vi "SubVI_GetIterNum.vi"(1 "#iter outer loop":i32, 2 "#iter inner loop":i32[](array[numeric]), 3 "N inner loop":i32) -> (0 "#iter GLOBAL":i32[](array[numeric]))   [LabVIEW 2018]
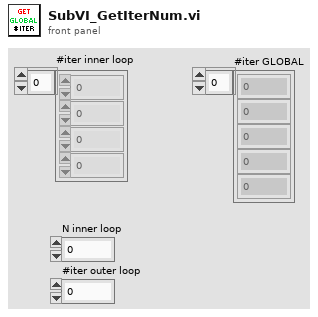
[diagram p1: front panel]
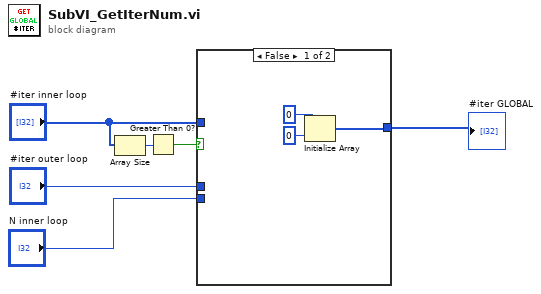
[diagram p0: block diagram]
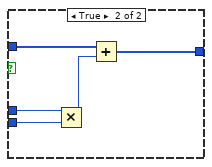
[diagram p2: hidden frame]
diagram:
  n1 = Array Size(array="#iter inner loop") -> (size(s)=w3:i32)
  n2 = Greater Than 0?(x=w3) -> (x > 0?=w2:bool)
  n3 = case shown="False" w2 {
    tunnel: [w7 w13] -> w6
    tunnel: "#iter inner loop" -> [_ w12]
    tunnel: "#iter outer loop" -> [_ w11]
    tunnel: "N inner loop" -> [_ w10]
    frame False {
      n4 = Initialize Array(0 ("element"), 0 ("dimension size")) -> (w7:i32[])
    }
    frame True {
      n5 = Multiply(x=w11, y=w10) -> (x*y=w14:i32)
      n6 = Add(x=w12, y=w14) -> (x+y=w13:i32[])
    }
  }
  "#iter GLOBAL" <- w6
